vi "Download Stats String.vi"(7 "Format String (3 floats)":string="%.1f / %.1f -- %.2f MB/s", 11 "Status Cluster":T1) -> (2 "Format Invalid":bool, 3 "Status String":string)   [LabVIEW 2018, in "HttpClient_NET.lvlib" / "HttpDownloadTask.lvclass"]
uses:
  HttpDownloadTask.lvclass
  Types/DownloadStats_Cluster.ctl
  HttpClient_NET.lvlib
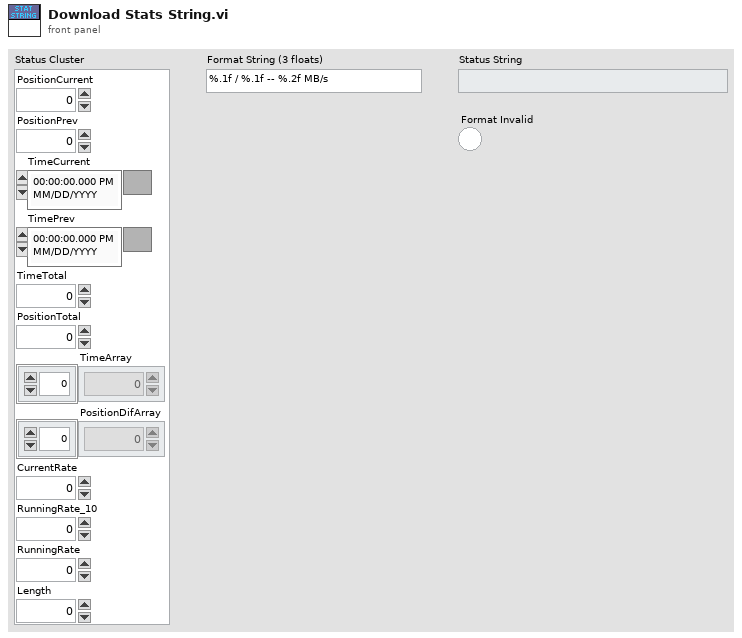
[diagram p1: front panel]
types:
  T1 = typedef "HttpClient_NET.lvlib/DownloadStats_Cluster.ctl" = cluster{"PositionCurrent":dbl, "PositionPrev":dbl, "TimeCurrent":timestamp, "TimePrev":timestamp, "TimeTotal":dbl, "PositionTotal":dbl, "TimeArray":dbl[], "PositionDifArray":dbl[], "CurrentRate":dbl, "RunningRate_10":dbl, "RunningRate":dbl, "Length":dbl}
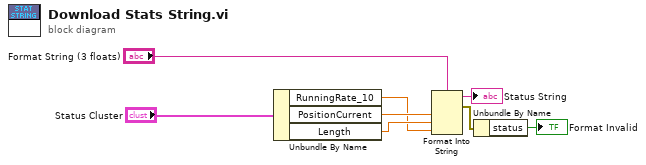
[diagram p0: block diagram]
diagram:
  n1 = Unbundle By Name("Status Cluster") -> ("RunningRate_10"=w6:dbl, "PositionCurrent"=w8:dbl, "Length"=w7:dbl)
  n2 = Format Into String(format string="Format String (3 floats)", w8, w7, w6) -> (resulting string=→"Status String":string, error out=w2:errorcluster)  [unwired: 2 in]
  n3 = Unbundle By Name(w2) -> ("status"=→"Format Invalid":bool)
